vi "子界面-查看某框和报告生成.vi"(0 "框号":dbl format="%#_13g", 1 "框组":T3(array[cluster]), 2 "标注图":T5(plugin-control), 3 "条件1-面积判断":T2(array[cluster]) {"Measurement Parameter" items=["Area"]; "下限" format="%.2f"; "上限" format="%.2f"}, 4 "条件2-灰度阈值":cluster{"下限":sgl, "上限":sgl}={"下限"=128.0, "上限"=255.0} {"下限" min=0 max=255 step=1; "上限" min=0 max=255 step=1}) -> ()   [LabVIEW 2018]
uses:
  <vilib>/vision/NI_Vision_Development_Module.lvlib
panel:
  in  "返回":bool
  in  "报告生成":bool
  in  "Color":u32[](array[colorbox])=[3381759, 16776770, 16777225, 6618880]
  in  "Overlay Type":u16[](array[ring])=[2, 1, 3, 0] items=["Rectangle", "Numbers", "Points", "Lines"]
  in  "Tab Control":T4
  out "原图":T5(plugin-control) caption="Original Image"
  out "阈值处理":T5(plugin-control) caption="Threshold Image"
  out "面积筛选":T5(plugin-control) caption="Reject Border and Fill Holes"
  out "缺陷统计":T5(plugin-control) caption="Filter Out Non Circles and Overlay Particle Area"
  out "灰度表":u32[](graph)
  out "最小灰度值":sgl
  out "最大灰度值":sgl
  out "平均值":sgl
  out "标准差":sgl
  out "Particle Measurements (Pixels)":dbl[][](array[numeric]) format="%.2f"
  in  "产品序号":string
  in  "测试人":string
  out "报告生成路径":path
  in  "分隔符（'\\'代码显示）":string="\t"
  in  "格式字符串":string="%f"
  out "缺陷检测结果":string[][](table)
  out "?":string
  out "面积 (pixels)":i32
  # "所选区域信息"
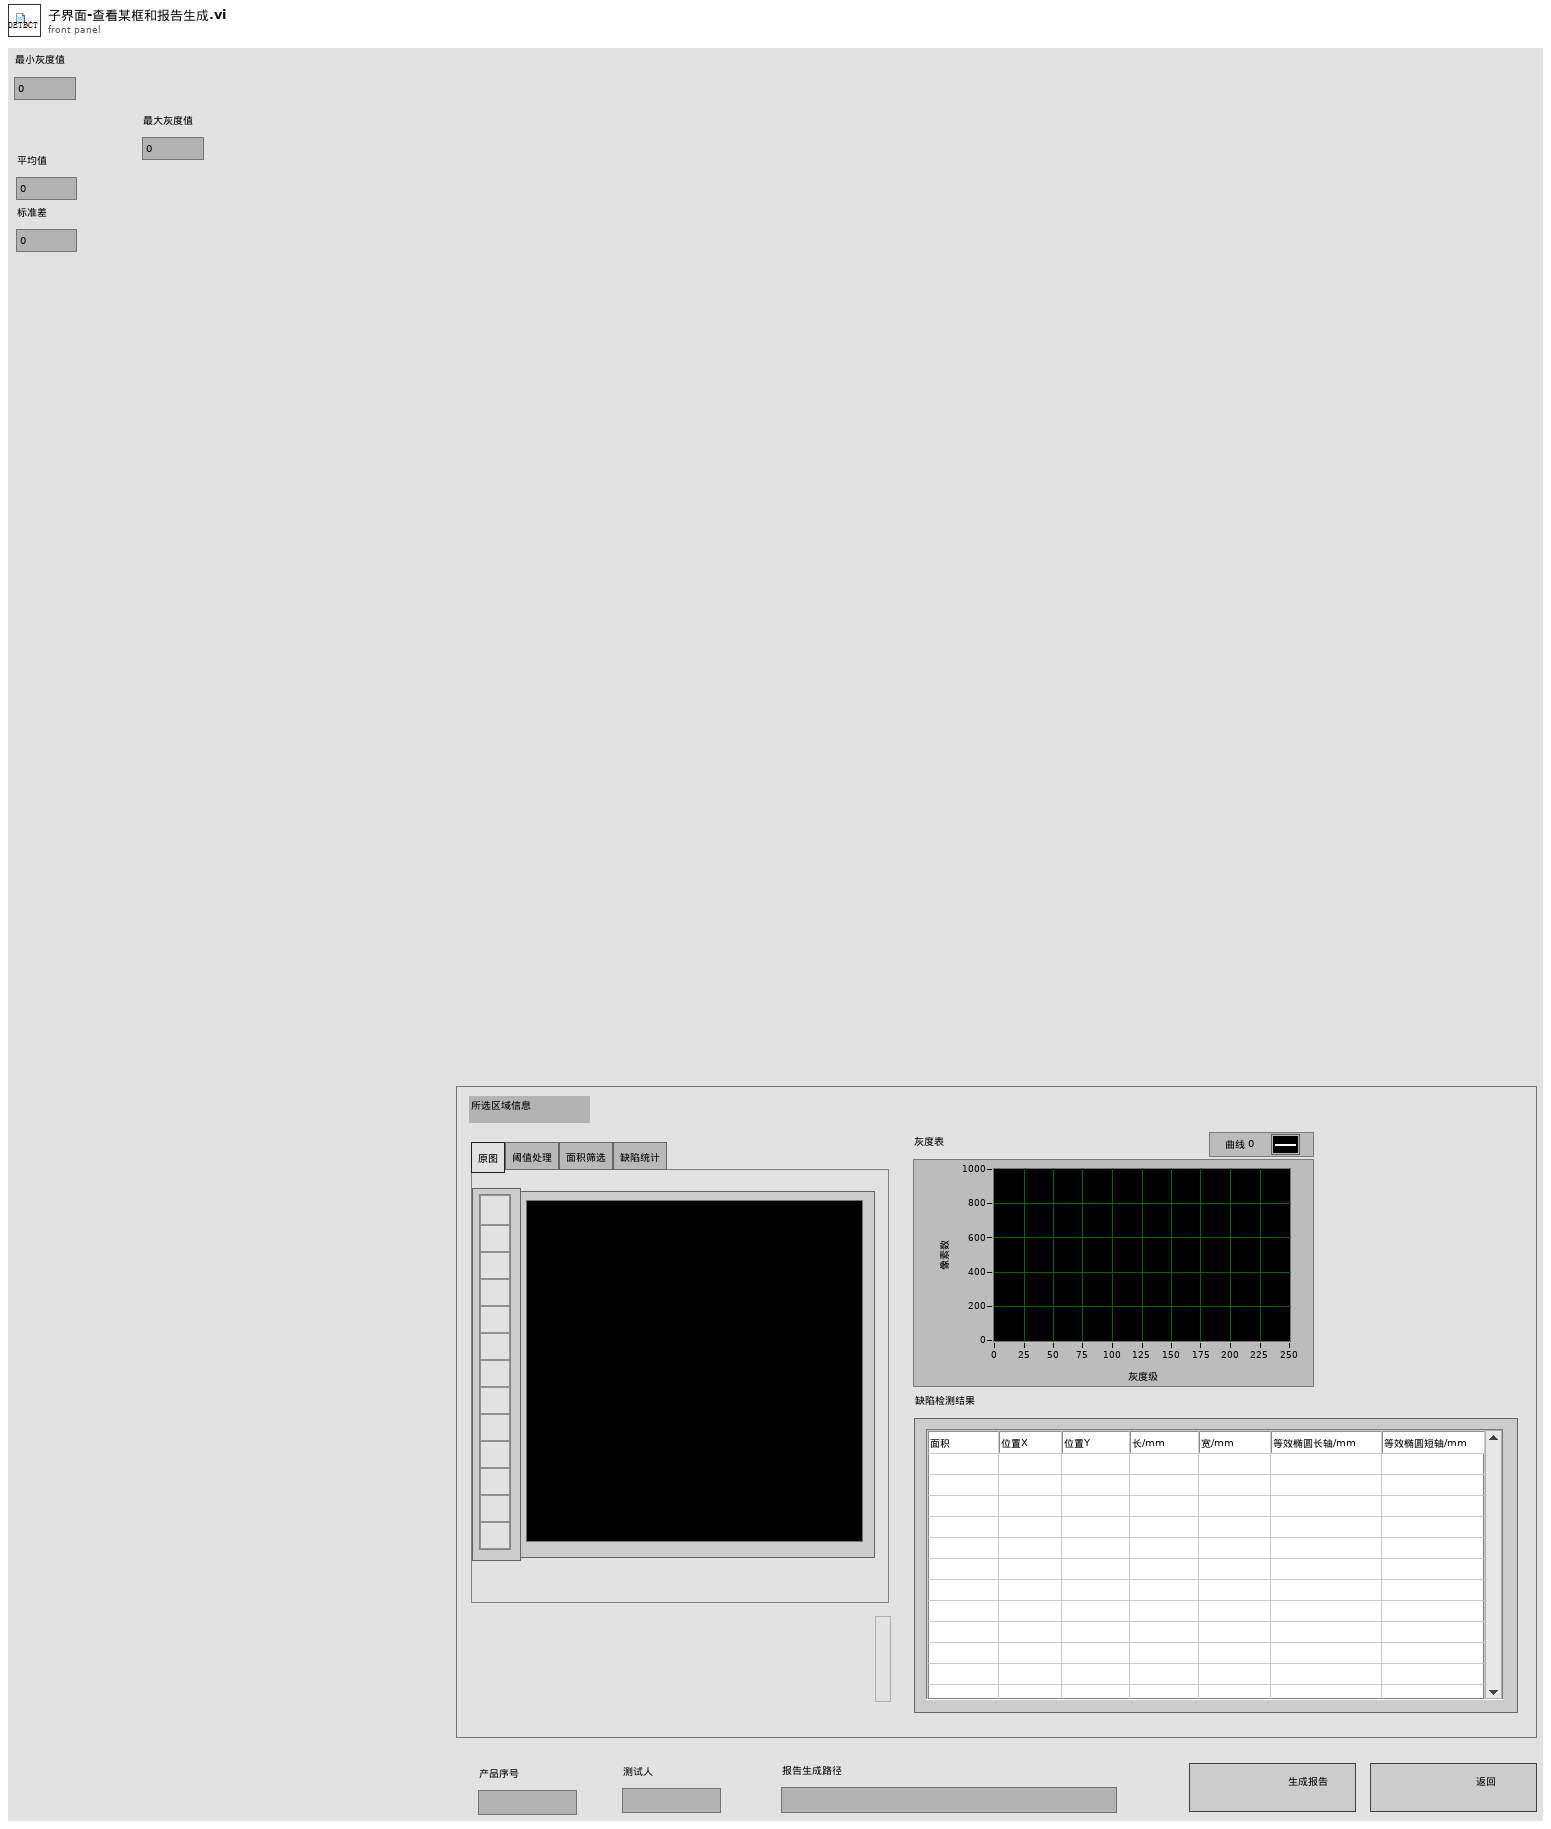
[diagram p1: front panel]
types:
  T1 = typedef "Particle Parameters" = i32
  T2 = cluster{"Measurement Parameter":T1, "下限":dbl, "上限":dbl, "Range":bool, "Measurement Type":bool}[]
  T3 = cluster{"Global Rectangle":i32[], "Contours":cluster{"Contour Type":u32, "ROI Type":u32, "Points":i32[]}[]}[]
  T4 = typedef "控件 1.ctl" = enum32{"原图", "阈值处理", "面积筛选", "缺陷统计"}
  T5 = typedef "IMAQ Image.ctl" = refnum<image>
  T6 = typedef "Image Type" = u32
  T7 = cluster{"Global Rectangle":i32[], "Contours":cluster{"Contour Type":u32, "ROI Type":u32, "Points":i32[]}[]}
  T8 = cluster{"条件2-灰度阈值":cluster{"下限":sgl, "上限":sgl}, "Pixel Measurements":T1[], "Overlay Type":u16[], "Color":u32[]}
  T9 = cluster{"histogram":u32[], "Minimal Value":sgl, "Maximal Value":sgl, "Starting Value":sgl, "Interval Width":sgl, "Mean Value":sgl, "Standard  Variation":sgl, "Area (pixels)":i32}
  T10 = cluster{"Desired Font (Application)":enum16{"User-specified Font", "Application Font", "System Font", "Dialog Font"}, "[User-specified Font]":cluster{"Font Name":string, "Size":i16, "Strikeout?":bool, "Italic?":bool, "Underline?":bool, "Outline?":bool, "Shadow?":bool, "Bold?":bool, "Rotation Angle":dbl}, "Horizontal Alignment":i16, "Vertical Alignment":i16}
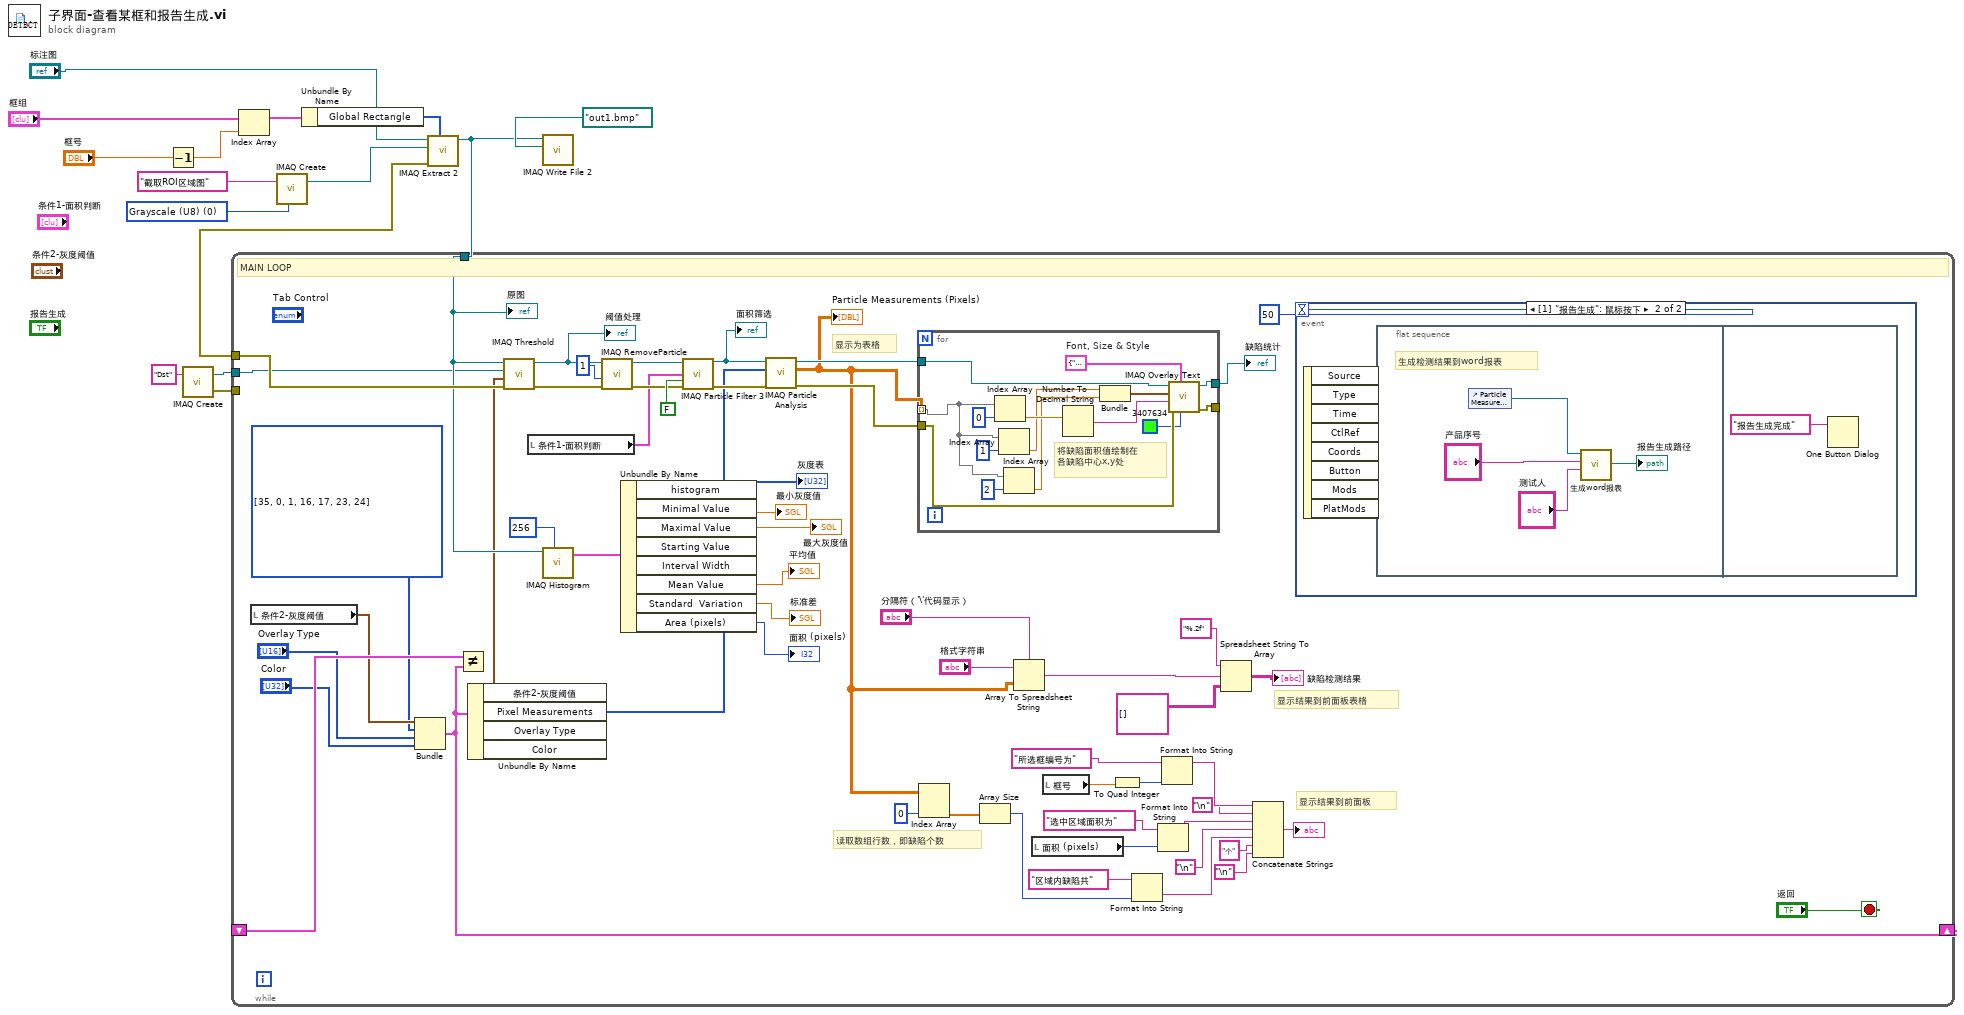
[diagram p0: block diagram]
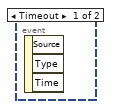
[diagram p2: hidden frame]
diagram:
  w13 = T6 0 items=["Grayscale (U8)", "Grayscale (I16)", "Grayscale (SGL)", "Complex (CSG)", "RGB (U32)", "HSL (U32)", "RGB (U64)", "Grayscale (U16)"] ("Image Type")
  n1 = Decrement(x="框号") -> (x-1=w15:dbl)
  n2 = call "IMAQ Create"("Image Name"="Dst") -> ("New Image"=w7:T5, "error out"=w6:errorcluster)  [unwired: 4 in]
  n3 = Index Array(array="框组", index=w15) -> (element=w10:T7)
  n4 = call "IMAQ Create"("Image Name"="截取ROI区域图", "Image Type"=w13) -> ("New Image"=w11:T5)  [unwired: 3 in, 1 out]
  n5 = Unbundle By Name(w10) -> ("Global Rectangle"=w14:i32[])
  n6 = call "IMAQ Extract 2"("Optional Rectangle"=w14, "Image Dst"=w11, "Image Src"="标注图") -> ("error out"=w5:errorcluster, "Image Dst Out"=w4:T5)  [unwired: 7 in]
  n7 = while "MAIN LOOP" {
    tunnel: w5 -> [w70]
    shift-right: [w71] -> _
    shift-left: _ -> [w72]
    tunnel: w7 -> [w41]
    tunnel: w6 -> [_]
    tunnel: w4 -> [w68]
    stop <- "返回" stop-if-true
    w64 = T1[] [35, 0, 1, 16, 17, 23, 24] items=["Center of Mass X", "Center of Mass Y", "First Pixel X", "First Pixel Y", "Bounding Rect Left", "Bounding Rect Top", "Bounding Rect Right", "Bounding Rect Bottom", "Max Feret Diameter Start X", "Max Feret Diameter Start Y", "Max Feret Diameter End X", "Max Feret Diameter End Y", "Max Horiz. Segment Length Left", "Max Horiz. Segment Length Right", "Max Horiz. Segment Length Row", "-", "Bounding Rect Width", "Bounding Rect Height", "Bounding Rect Diagonal", "Perimeter", "Convex Hull Perimeter", "Holes' Perimeter", "Max Feret Diameter", "Equivalent Ellipse Major Axis", "Equivalent Ellipse Minor Axis", "Equivalent Ellipse Minor Axis (Feret)", "Equivalent Rect Long Side", "Equivalent Rect Short Side", "Equivalent Rect Diagonal", "Equivalent Rect Short Side (Feret)", "Average Horiz. Segment Length", "Average Vert. Segment Length", "Hydraulic Radius", "Waddel Disk Diameter", "-", "Area", "Holes' Area", "Particle & Holes' Area", "Convex Hull Area", "Image Area", "-", "Number of Holes", "Number of Horiz. Segments", "Number of Vert. Segments", "-", "Orientation", "Max Feret Diameter Orientation", "-", "% Area/Image Area", "% Area/(Particle & Holes' Area)", "Ratio of Equivalent Ellipse Axes", "Ratio of Equivalent Rect Sides", "-", "Elongation Factor", "Compactness Factor", "Heywood Circularity Factor", "Type Factor", "-", "Sum X", "Sum Y", "Sum XX", "Sum XY", "Sum YY", "Sum XXX", "Sum XXY", "Sum XYY", "Sum YYY", "-", "Moment of Inertia XX", "Moment of Inertia XY", "Moment of Inertia YY", "Moment of Inertia XXX", "Moment of Inertia XXY", "Moment of Inertia XYY", "Moment of Inertia YYY", "Norm. Moment of Inertia XX", "Norm. Moment of Inertia XY", "Norm. Moment of Inertia YY", "Norm. Moment of Inertia XXX", "Norm. Moment of Inertia XXY", "Norm. Moment of Inertia XYY", "Norm. Moment of Inertia YYY", "Hu Moment 1", "Hu Moment 2", "Hu Moment 3", "Hu Moment 4", "Hu Moment 5", "Hu Moment 6", "Hu Moment 7"] ("Pixel Measurements")
    # "显示结果到前面板"
    # "读取数组行数，即缺陷个数"
    # "显示结果到前面板表格"
    # "显示为表格"
    # "MAIN LOOP"
    n8 = local read "条件2-灰度阈值"() -> (w65:cluster{"下限":sgl, "上限":sgl})
    n9 = Bundle("条件2-灰度阈值"=w65, "Pixel Measurements"=w64, "Overlay Type"="Overlay Type", "Color"="Color") -> (w71:T8)  [unwired: 1 in]
    n10 = Not Equal?(x=w72, y=w71) -> ()  [unwired: 1 out]
    n11 = Unbundle By Name(w71) -> ("条件2-灰度阈值"=w55:cluster{"下限":sgl, "上限":sgl}, "Pixel Measurements"=w54:T1[])  [unwired: 2 out]
    n12 = call "IMAQ Threshold"("error in (no error)"=w70, "Range"=w55, "Image Dst"=w41, "Image Src"=w68) -> ("error out"=w60:errorcluster, "Image Dst Out"=w46:T5)  [unwired: 2 in, 4 out]
    "阈值处理" <- w46
    n13 = local read "条件1-面积判断"() -> (w44:T2)
    n14 = call "IMAQ Histogram"("Number of Classes"=256, "Image"=w68) -> ("Histogram Report"=w48:T9)  [unwired: 8 in, 1 out]
    n15 = call "IMAQ RemoveParticle"("error in (no error)"=w60, "Number of Erosion"=1, "Image Src"=w46) -> ("error out"=w59:errorcluster, "Image Dst Out"=w62:T5)  [unwired: 7 in]
    n16 = Unbundle By Name(w48) -> ("histogram"=→"灰度表":u32[], "Minimal Value"=→"最小灰度值":sgl, "Maximal Value"=→"最大灰度值":sgl, "Mean Value"=→"平均值":sgl, "Standard  Variation"=→"标准差":sgl, "Area (pixels)"=→"面积 (pixels)":i32)  [unwired: 2 out]
    n17 = call "IMAQ Particle Filter 3"("Image Src"=w62, "Selection Values"=w44, "Keep/Remove Particles (F)"=FALSE, "error in (no error)"=w59) -> ("Image Dst Out"=w45:T5, "error out"=w58:errorcluster)  [unwired: 9 in, 1 out]
    "面积筛选" <- w45
    n18 = call "IMAQ Particle Analysis"("error in (no error)"=w58, "Pixel Measurements"=w54, "Image"=w45) -> ("error out"=w56:errorcluster, "Particle Measurements (Pixels)"=w16:dbl[][], "Image Out (duplicate)"=w57:T5)  [unwired: 3 in, 3 out]
    "Particle Measurements (Pixels)" <- w16
    n19 = for {
      tunnel: w56 -> [w92]
      tunnel: [w91] -> _
      tunnel: [w90] -> w69
      tunnel: w57 -> [w88]
      tunnel: w16 -> [w80] mode=indexing
      w87 = T10 {"Desired Font (Application)"=enum."Application Font", "[User-specified Font]"={"Font Name"="", "Size"=12, "Strikeout?"=FALSE, "Italic?"=FALSE, "Underline?"=FALSE, "Outline?"=FALSE, "Shadow?"=FALSE, "Bold?"=FALSE, "Rotation Angle"=0.0}, "Horizontal Alignment"=0, "Vertical Alignment"=0}  # Font, Size & Style
      # "将缺陷面积值绘制在\n各缺陷中心x,y处"
      n20 = Index Array(array=w80, index=0 ("索引")) -> (element=w85:dbl)
      n21 = Index Array(array=w80, index=1 ("索引")) -> (element=w82:dbl)
      n22 = Index Array(array=w80, index=2 ("索引")) -> (element=w79:dbl)
      n23 = Number To Decimal String(number=w85) -> (decimal integer string=w86:string)  [unwired: 1 in]
      n24 = Bundle("Numeric"=w82, "Numeric"=w79) -> (w78:cluster{"Numeric":dbl, "Numeric":dbl})  [unwired: 1 in]
      n25 = call "IMAQ Overlay Text"("Text Color (black)"=u32 3407634, "Font, Size & Style"=w87, "error in (no error)"=w92, "String"=w86, "Origin"=w78, "Image"=w88) -> ("error out"=w91:errorcluster, "Image Out"=w90:T5)  [unwired: 4 in]
    }
    "缺陷统计" <- w69
    n26 = Index Array(array=w16, index (col)=0 ("禁用的索引 (列)")) -> (element=w27:dbl[])  [unwired: 1 in]
    n27 = Array Size(array=w27) -> (size(s)=w29:i32)
    n28 = Array To Spreadsheet String(delimiter (Tab)="分隔符（'\\'代码显示）", array=w16, 3:"格式字符串") -> (spreadsheet string=w37:string)
    n29 = local read "面积 (pixels)"() -> (w26:i32)
    n30 = local read "框号"() -> (w31:dbl)
    n31 = To Quad Integer(1:w31) -> (0:w30:i64)
    n32 = Format Into String(initial string="区域内缺陷共" ("初始字符串"), w29) -> (resulting string=w33:string)  [unwired: 2 in, 1 out]
    n33 = Format Into String(initial string="选中区域面积为" ("字符串"), w26) -> (resulting string=w34:string)  [unwired: 2 in, 1 out]
    n34 = Format Into String(initial string="所选框编号为" ("初始字符串"), w30) -> (resulting string=w32:string)  [unwired: 2 in, 1 out]
    n35 = Spreadsheet String To Array(format string="%.2f", spreadsheet string=w37, array type (2D Dbl)=string[][] [] ("Array")) -> (array=→"缺陷检测结果":string[][])  [unwired: 1 in]
    n36 = Concatenate Strings(w32, "\n", w34, "\n", w33, "个" ("字符串"), "\n") -> (→"?":string)
    n37 = event shown="[1] \"报告生成\": 鼠标按下" {
      selector: _ -> [_ _]
      dyn-events: _ -> [_ _]
      timeout: 50 -> [_ _]
      event Timeout {
        n38 = event-data() -> ()  [unwired: 1 in, 3 out]
      }
      event "报告生成": Mouse Down {
        n39 = event-data() -> ()  [unwired: 1 in, 8 out]
        n40 = flat-sequence {
          frame #0 {
            # "生成检测结果到word报表"
            n41 = control-ref of="Particle Measurements (Pixels)"() -> (w74:refnum<vi>)
            n42 = call "生成word报表.vi"("测试人"="测试人", "产品序号"="产品序号", "Array输入"=w74) -> ("报告生成路径"=→"报告生成路径":path)  [unwired: 8 in]
          }
          frame #1 {
            n43 = One Button Dialog(message="报告生成完成" ("消息")) -> ()  [unwired: 1 in, 1 out]
          }
        }
      }
    }
    "原图" <- w68
  }
  n44 = call-poly "IMAQ Write File 2"("File Path"=path "out1.bmp", "Image"=w4) -> ()  [unwired: 8 in, 2 out]
